vi "PDF_Interface_PDF Protokoll EPA1065_308 T90.vi"(8 "error in (no error)":errorcluster caption="Fehler (Eingang, kein Fehler)", 9 "ResultPictures":T1, 10 "SVGraph Referenz":refnum<vi>, 11 "Save PDF File Path":path) -> (0 "error out":errorcluster caption="Fehler (Ausgang)")   [LabVIEW 2020, in "EPA 1065.lvlib" / "T90 Test 1065-308.lvlib"]
uses:
  T90 Test 1065-308.lvlib
  Ergebnis.ctl
  PDF_Interface/PDF Interface Helper/PDFResultPictures.ctl
  Sprachverwaltung/FGV Aktion Tabelle zerlegen.ctl
  Aktion FGV T90.ctl
  Seiten/FT-IR/FGV FT-IR Gasliste Aktionen.ctl
  Seiten/FT-IR/FGV FT-IR Aktionen.ctl
  Seiten/System Einstellungen V2/Aktioen FGV System Konstanten.ctl
  PDF_Interface/PDF Protokoll Standard Kopf Optionen.ctl
  Visualisierungs Elemente/Auswahlfeld.ctl
  PDF_Interface/PDF Protokoll Standard Kopf Gasflasche Auswahl.ctl
  Aktion FGV Datenmanagment.ctl
  PDF_Interface/PDF Interface Helper/PDFGraph.ctl
  <vilib>/Simplicity AI/SAI_PDF_API/Classes/Context/Controls/SAI_PDF_Text Align.ctl
  PDF_Interface/PDF Interface Helper/PDFCommentPosition.ctl
  PDF_Interface/PDF Interface Helper/PDFPageBreak.ctl
  <vilib>/Simplicity AI/SAI_PDF_API/Classes/Context/Controls/SAI_PDF_PDF Details.ctl
  PDF_Interface/PDF Interface Helper/PDFContentType.ctl
  PDF_Interface/PDF Interface Helper/PDFTableContentType.ctl
  PDF_Interface/PDF Interface Helper/PDFResults.ctl
  PDF_Interface/PDF Interface Helper/PDFTablePictures.ctl
  PDF_Interface/PDF Interface Helper/PDFBemerkung.ctl
  <vilib>/Simplicity AI/SAI_PDF_API/Classes/Context/Controls/SAI_PDF_Font.ctl
  <vilib>/Simplicity AI/SAI_PDF_API/Classes/Context/Controls/SAI_PDF_Font Encoding.ctl
  Allgemein/allgemeine Sub-VIs.lvlib
  Seiten/FT-IR/FT-IR.lvlib
  Seiten/System Einstellungen V2/System Einstellungen V2.lvlib
  Sprachverwaltung/Sprachverwaltung.lvlib
  PDF_Interface/PDF Interface.lvlib
  PDF_Interface/PDF Interface Helper/PDF Interface Helper.lvlib
  <vilib>/Simplicity AI/SAI_PDF_API/Classes/Context/Context.lvclass
  Linearisierung V2/Protokoll/Protokoll.lvlib
panel:
  out "Frequenz 2":string
  out "Frequenz 1":string
  out "Versa Serial number:":string caption="Seriennummer:"
  out "Anlage:":string
  out "Methode (Recipe):":string
  out "Date & Time:":string caption="Datum & Uhrzeit:"
  out "Accuracy:":string caption="Genauigkeit:"
  out "Gas Bottle Nr.:":string caption="Gasflaschen Nr.:"
  out "Ergebnis 4":T2
  out "Ergebnis 3":T2
  out "Ergebnis 2":T2
  out "Ergebnis 1":T2
  out "Averaged T90-T10 2":string caption="gemittelter T90-T10"
  out "Averaged T10-T90 2":string caption="gemittelter T10-T90"
  out "Ergebnis x5 (T90 T10)":string caption="Mean T10-T90"
  out "Ergebnis x5 (T10 T90)":string caption="Mean T10-T90"
  out "Averaged T90-T10":string caption="gemittelter T90-T10"
  out "Averaged T10-T90":string caption="gemittelter T10-T90"
  out "T90 Result":waveform(sgl)(graph) caption="T90"
  out "Tabelle":string[][](table)
  out "Ergebnis:":string
  out "Konzentration:":string
  out "Komponente:":string
  out "Bearbeiter:":string caption="Editor:"
  out "Serial number:":string caption="Seriennummer:"
  out "Messgerät:":string
  # "T90 EPA § 1065.308"
  # "Grenzen"
  # "Ergebnis"
  # "s"
  # ">5"
  # "s"
  # ">5"
  # "s"
  # "<10s"
  # "s"
  # "<10s"
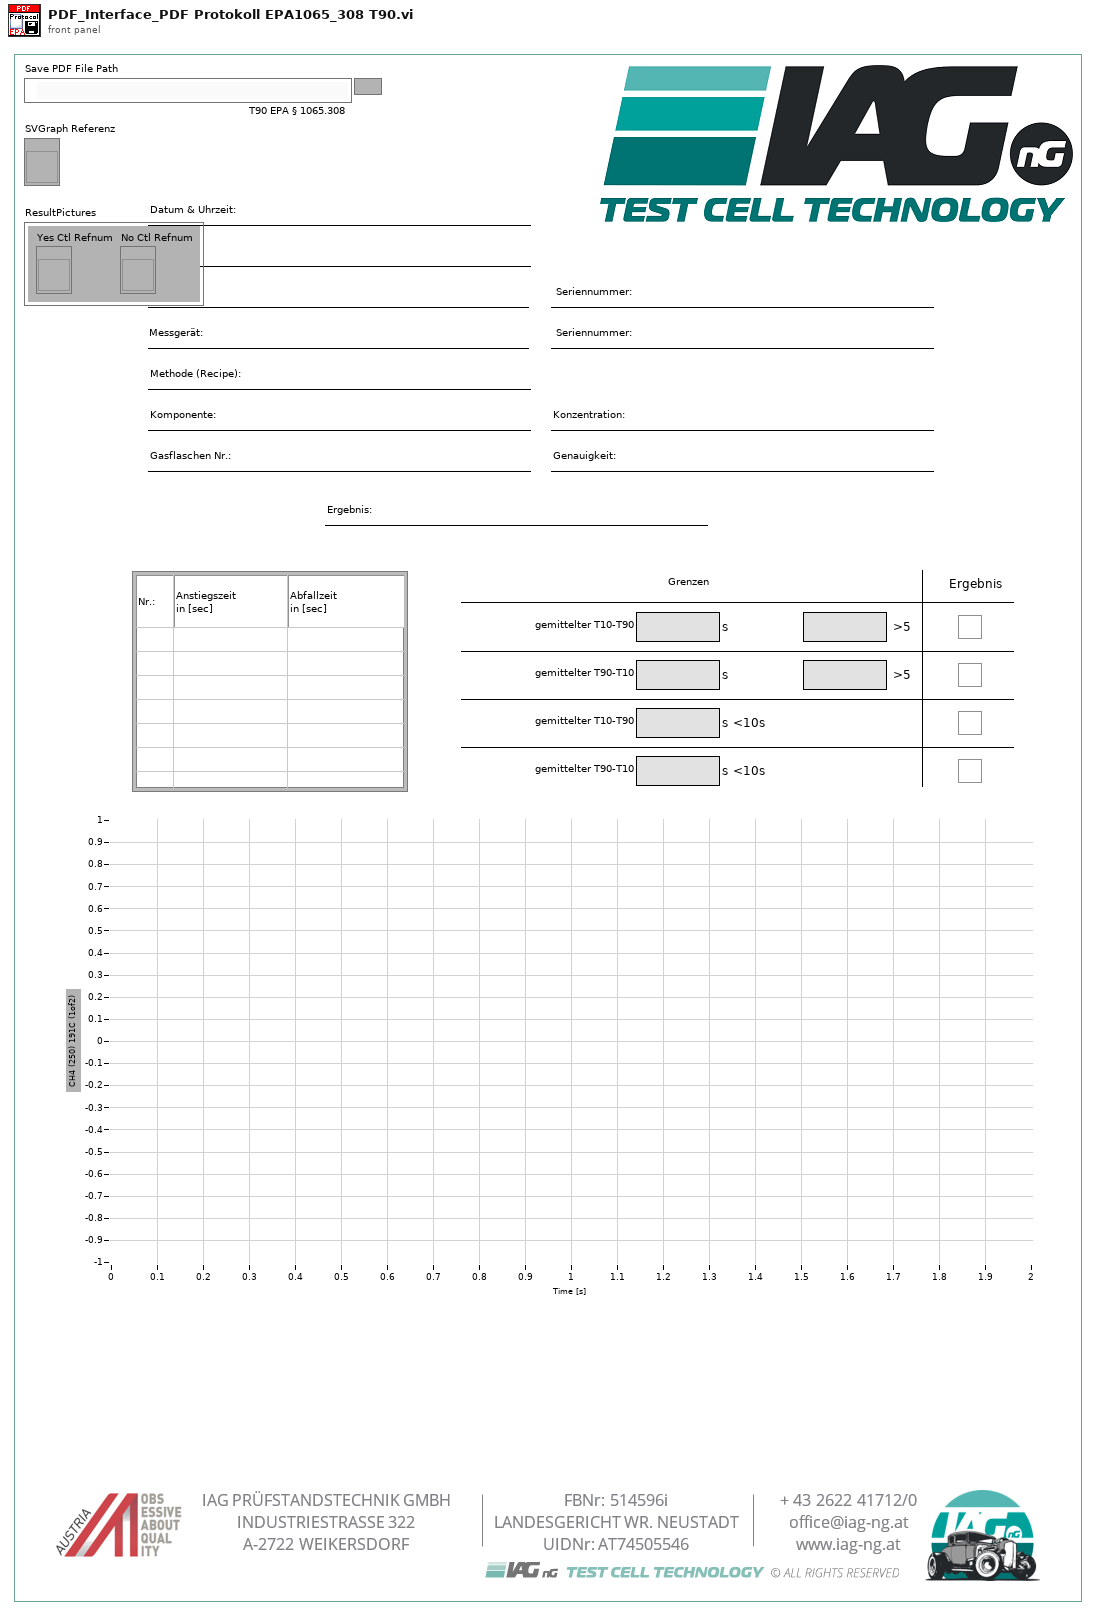
[diagram p1: front panel]
types:
  T1 = typedef "PDF Interface.lvlib/PDF Interface Helper.lvlib/PDFResultPictures.ctl" = cluster{"Yes Ctl Refnum":refnum<vi>, "No Ctl Refnum":refnum<vi>}
  T2 = typedef "EPA 1065.lvlib/T90 Test 1065-308.lvlib/Ergebnis.ctl" = bool
  T3 = typedef "Sprachverwaltung.lvlib/FGV Aktion Tabelle zerlegen.ctl" = enum16{"laden", "vereinzeln", "speichern"}
  T4 = typedef "PDF Interface.lvlib/PDF Protokoll Standard Kopf Gasflasche Auswahl.ctl" = cluster{"Gasflaschen Name":string, "Gasflaschen Nummer":string, "Gasnummer Index":i32}
  T5 = typedef "Auswahlfeld.ctl" = u16
  T6 = typedef "PDF Interface.lvlib/PDF Protokoll Standard Kopf Optionen.ctl" = cluster{"Analysator":bool, "FT-IR Rezept":bool, "Gasteiler":bool, "Gas Komponente":bool, "Gas Flasche":bool, "LIN Protokoll":bool, "Operator":bool}
  T7 = typedef "System Einstellungen V2.lvlib/Aktioen FGV System Konstanten.ctl" = enum16{"lesen", "laden", "speichern", "Sprache"}
  T8 = typedef "FT-IR.lvlib/FGV FT-IR Aktionen.ctl" = enum16{"lesen", "NOG setzen", "NOS setzen", "Initialisieren", "speichern", "ALLES setzen", "FT-IR Spektrum loggen", "Komm Stoppen", "Spektrum LogKonfig"}
  T9 = typedef "FT-IR.lvlib/FGV FT-IR Gasliste Aktionen.ctl" = enum16{"lesen", "Gasliste FT-IR", "Gasliste ausgelesen", "laden", "speichern", "löschen"}
  T10 = typedef "EPA 1065.lvlib/T90 Test 1065-308.lvlib/Aktion FGV T90.ctl" = enum16{"lesen", "Konfig Daten", "speichern", "laden", "T90 aktiv", "T90 inaktiv", "Ext. Ventil aktivieren", "Ext. Ventil deaktivieren", "N2 spülen aktiv", "N2 spülen inaktiv", "Ergebnis Textfile"}
  T11 = typedef "EPA 1065.lvlib/T90 Test 1065-308.lvlib/Aktion FGV Datenmanagment.ctl" = enum16{"init", "lesen", "Istwerte schreiben", "höchsten Peak setzen", "Auswerten", "Grenzen setzen", "Sollwert ändern", "Rise T10", "Rise T90", "Fall T90", "Fall T10", "Bit löschen", "Umschaltzeitpunkt"}
  T12 = typedef "PDF Interface.lvlib/PDF Interface Helper.lvlib/PDFBemerkung.ctl" = cluster{"Bemerkung Text":string, "Align (Left)":T13, "Add Line Feeds (F:No)":bool, "Font":T14}
  T13 = typedef "SAI_PDF_Toolkit.lvlib/Context.lvclass/SAI_PDF_Text Align.ctl" = i32
  T14 = typedef "SAI_PDF_Toolkit.lvlib/Context.lvclass/SAI_PDF_Font.ctl" = cluster{"Font":string, "Size":i32, "Colour":u32, "Bold":bool, "Italic":bool, "Underline":bool, "Strikethrough":bool, "Font Encoding":T15}
  T15 = typedef "SAI_PDF_Toolkit.lvlib/Context.lvclass/SAI_PDF_Font Encoding.ctl" = enum16{"Cp1252, WinANSI", "IdentityH", "IdentityV", "Cp1250", "Cp1257", "MacRoman"}
  T16 = typedef "PDF Interface.lvlib/PDF Interface Helper.lvlib/PDFContentType.ctl" = cluster{"Titel":string, "Header Table":string[][], "Table Array":T17[], "Bemerkungen":T12[]}
  T17 = typedef "PDF Interface.lvlib/PDF Interface Helper.lvlib/PDFTableContentType.ctl" = cluster{"TableHeader":string[], "Table":string[][], "Relative Column Widths (%)":sgl[], "Results":T18, "PositionBemerkung":T19, "PageBreak":T20, "TablePictures":T21, "Horizontal Align":i32}
  T18 = typedef "PDF Interface.lvlib/PDF Interface Helper.lvlib/PDFResults.ctl" = cluster{"Results":cluster{"Result Text":string, "Result":bool}[], "ResultPictures":T1, "use Pictures":bool, "Image Scale (%)":sgl, "Autoscale? (T)":bool, "Horizontal Align":i32, "Position":i32}
  T19 = typedef "PDF Interface.lvlib/PDF Interface Helper.lvlib/PDFCommentPosition.ctl" = enum16{"before", "after"}
  T20 = typedef "PDF Interface.lvlib/PDF Interface Helper.lvlib/PDFPageBreak.ctl" = enum16{"none", "before", "after", "after comment"}
  T21 = typedef "PDF Interface.lvlib/PDF Interface Helper.lvlib/PDFTablePictures.ctl" = cluster{"Ctl Refnum In":refnum<vi>[], "RowOrColumn":enum16{"Row", "Column"}, "IndexToInsert":u16, "Image Scale (%)":sgl[], "Autoscale? (T)":bool[], "Horizontal Align":i32}
  T22 = typedef "SAI_PDF_Toolkit.lvlib/Context.lvclass/SAI_PDF_PDF Details.ctl" = cluster{"Title":string, "Subject":string, "Keywords":string, "Author":string, "Creator":string}
  T23 = cluster{"Header Footer Text Cluster":cluster{"Header Text":string, "Footer Text":string, "Time":string, "Page Number":string}, "PDF Details":T22}
  T24 = typedef "EPA 1065.lvlib/T90 Test 1065-308.lvlib/T90 Konfig Daten.ctl" = cluster{"Bearbeiter:":string, "Komponente:":u16, "Gasflaschen Nr.:":string, "Accuracy":dbl, "Sollwert":dbl, "Modus":T25, "Abschaltzeit:":dbl, "Abweichung:":dbl, "Pfad:":path, "Textname:":string, "CG Aufschaltzeit:":dbl, "Einheit":string, "N2 Aufschaltzeit:":dbl, "Analysator":T26, "Gasflasche":T27, "Konfig Gasflasche":T28, "Frequency:":T29}
  T25 = typedef "EPA 1065.lvlib/T90 Test 1065-308.lvlib/Modus.ctl" = u16
  T26 = typedef "System Einstellungen V2.lvlib/Analysatoren.ctl" = string
  T27 = typedef "System Einstellungen V2.lvlib/Gasflasche Auswahl.ctl" = u16
  T28 = typedef "System Einstellungen V2.lvlib/Konfig Gasflasche.ctl" = bool
  T29 = typedef "EPA 1065.lvlib/T90 Test 1065-308.lvlib/Frequenz.ctl" = u16
  T30 = typedef "String - Ausgabefeld.ctl" = string
  T31 = cluster{"Header Size":i32, "Column Ratio left":sgl[]}
  T32 = cluster{"Modell":string, "ProjektNummer":string, "Software Version":string, "Seriennummer":string}
  T33 = typedef "EPA 1065.lvlib/T90 Test 1065-308.lvlib/Datencluster.ctl" = cluster{"Höchster Peak":T34, "T10 Grenzwert":T34, "T90 Grenzwert":T34, "Rise Times":dbl[], "Fall Times":dbl[], "RiseTime gemittelt":T34, "FallTime gemittelt":T34, "Zeitstempel":timestamp[], "Rise T10":bool, "Rise T90":bool, "Fall T10":bool, "Fall T90":bool, "RiseTime >5":bool, "Falltime >5":bool, "RiseTime <10":bool, "Falltime <10":bool, "T0-T90":dbl[], "T100-T10":dbl[]}
  T34 = typedef "Zahlen-Eingabefeld.ctl" = sgl
  T35 = typedef "PDF Interface.lvlib/PDF Interface Helper.lvlib/PDFGraph.ctl" = cluster{"GraphCtl Refnum":refnum<vi>, "Wrap Text (F:No)":bool, "Hide Grid (F:No)":bool, "Scale (100%)":sgl, "Align (Left)":T13, "PositionBemerkung":T19, "PageBreak":T20}
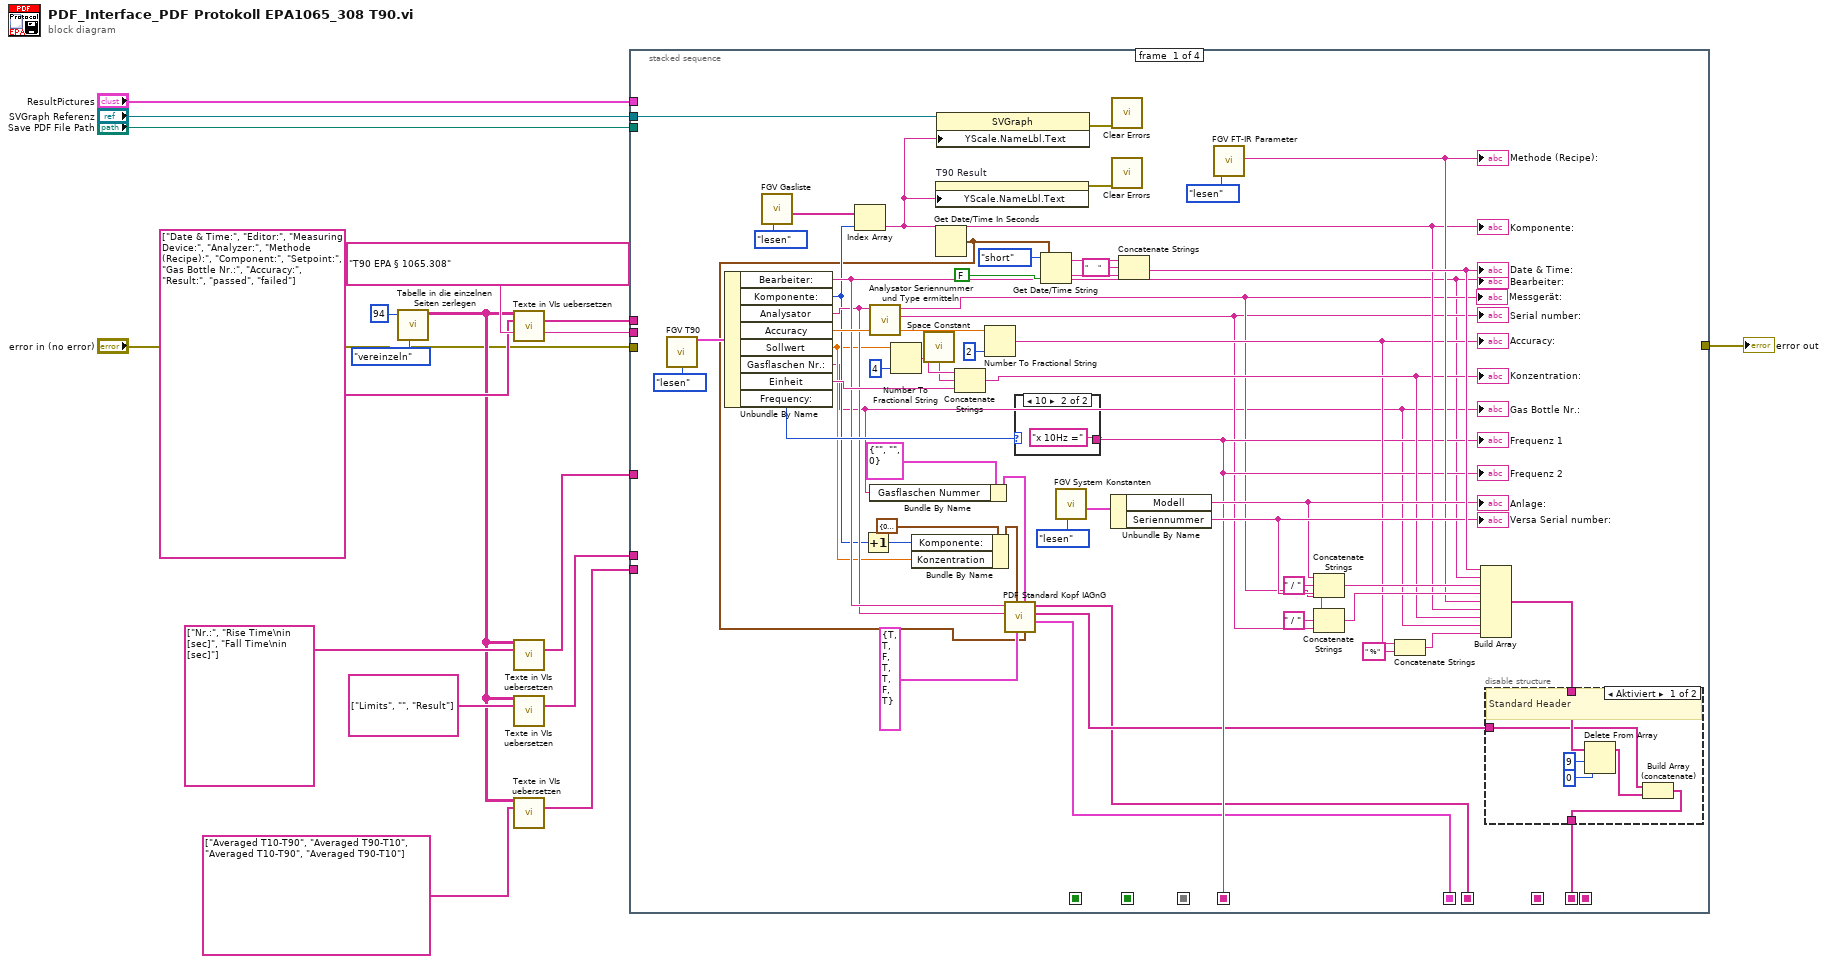
[diagram p0: block diagram]
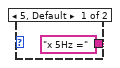
[diagram p3: hidden frame]
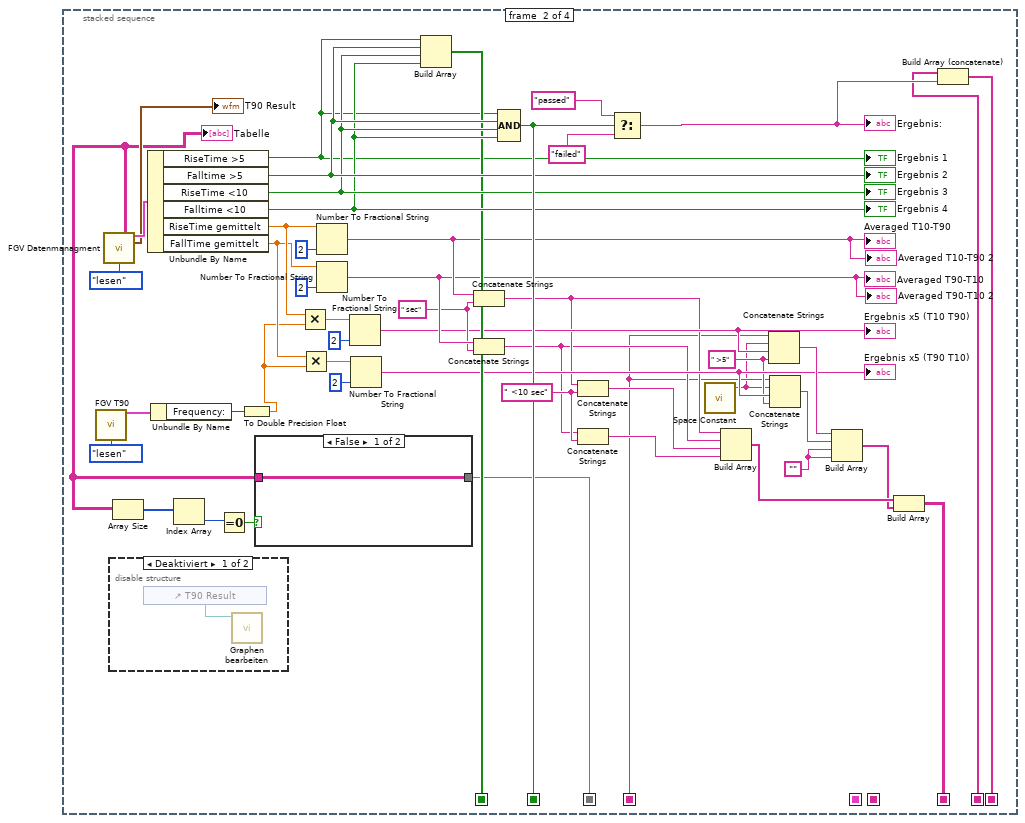
[diagram p4: hidden frame]
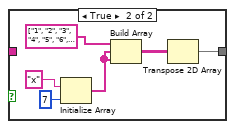
[diagram p5: hidden frame]
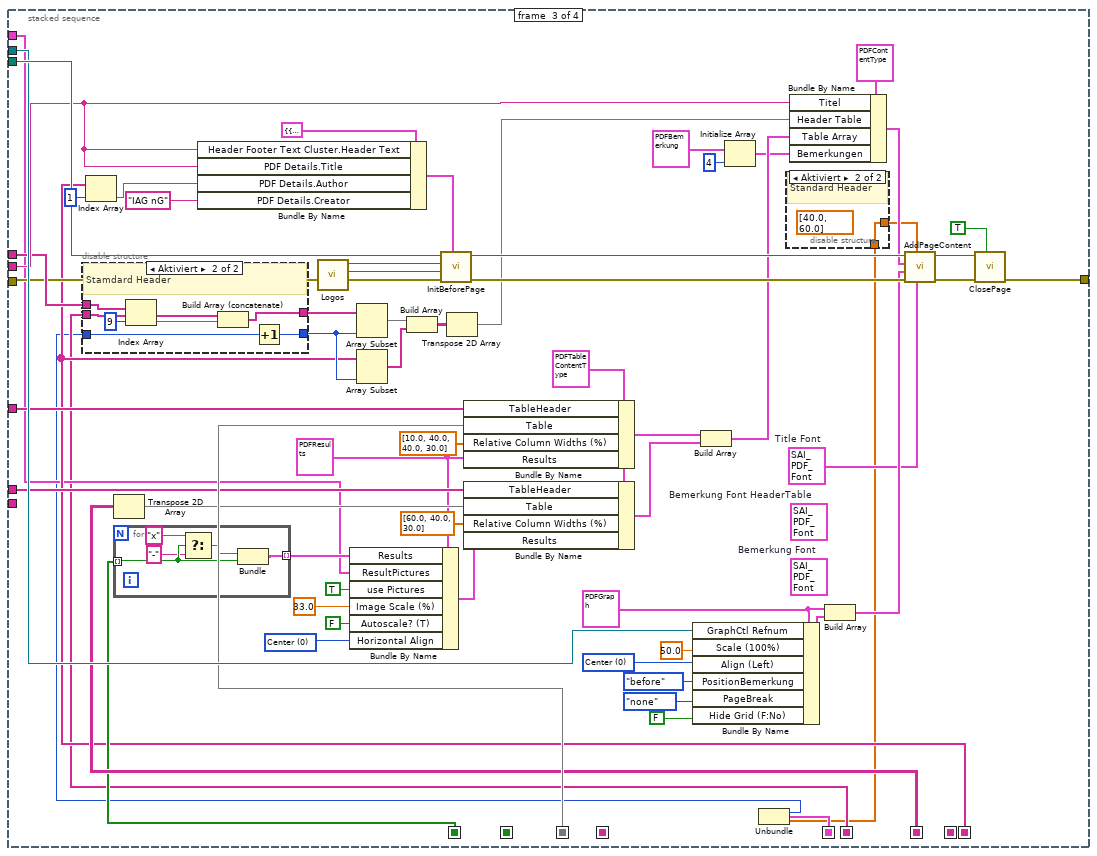
[diagram p7: hidden frame]
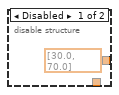
[diagram p8: hidden frame]
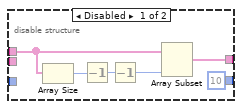
[diagram p9: hidden frame]
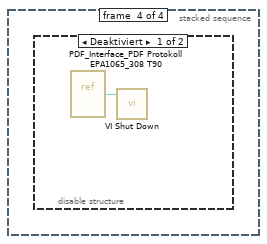
[diagram p10: hidden frame]
diagram:
  n1 = call "Tabelle in die einzelnen Seiten zerlegen.vi"("Aktion"=FGV_Aktion_Tabelle_zerlegen."vereinzeln", "Index (Seite)"=94) -> ("Sprachliste"=w8:string[][])  [unwired: 7 in, 2 out]
  n2 = call "Texte in VIs uebersetzen.vi"("Sprachliste"=w8, "String-Array zum Übersetzen"=string[] ["Date & Time:", "Editor:", "Measuring Device:", "Analyzer:", "Methode (Recipe):", "Component:", "Setpoint:", "Gas Bottle Nr.:", "Accuracy:", "Result:", "passed", "failed"], "String zum Übersetzen"="T90 EPA § 1065.308") -> ("String-Array zum Übersetzen"=w13:string[], "String zum Übersetzen"=w14:string)  [unwired: 8 in, 3 out]
  n3 = call "Texte in VIs uebersetzen.vi"("Sprachliste"=w8, "String-Array zum Übersetzen"=string[] ["Nr.:", "Rise Time\nin [sec]", "Fall Time\nin [sec]"]) -> ("String-Array zum Übersetzen"=w6:string[])  [unwired: 9 in, 4 out]
  n4 = call "Texte in VIs uebersetzen.vi"("Sprachliste"=w8, "String-Array zum Übersetzen"=string[] ["Limits", "", "Result"]) -> ("String-Array zum Übersetzen"=w5:string[])  [unwired: 9 in, 4 out]
  n5 = call "Texte in VIs uebersetzen.vi"("Sprachliste"=w8, "String-Array zum Übersetzen"=string[] ["Averaged T10-T90", "Averaged T90-T10", "Averaged T10-T90", "Averaged T90-T10"]) -> ("String-Array zum Übersetzen"=w4:string[])  [unwired: 9 in, 4 out]
  n6 = stacked-sequence {
    seq-local: [_ w86 _ _] -> [_ _ w166 _]
    seq-local: [_ w115 _ _] -> [_ _ _ _]
    seq-local: [_ w111 _ _] -> [_ _ w160 _]
    seq-local: [w23 _ _ _] -> [_ w109 _ _]
    seq-local: [_ w108 _ _] -> [_ _ w155 _]
    seq-local: [_ w91 _ _] -> [_ _ w161 _]
    seq-local: [w38 _ _ _] -> [_ w85 _ _]
    seq-local: [w22 _ _ _] -> [_ _ w144 _]
    seq-local: [w21 _ _ _] -> [_ _ w143 _]
    tunnel: w14 -> [_ _ w170 _]
    tunnel: w13 -> [_ _ w169 _]
    tunnel: "Save PDF File Path" -> [_ _ w172 _]
    tunnel: "SVGraph Referenz" -> [w54 _ w171 _]
    tunnel: w6 -> [_ _ w165 _]
    tunnel: w5 -> [_ _ w163 _]
    tunnel: w4 -> [_ _ _ _]
    tunnel: "error in (no error)" -> [_ _ w168 _]
    tunnel: [_ _ w167 _] -> w2
    tunnel: "ResultPictures" -> [_ _ w150 _]
    frame #0 {
      n7 = call "FGV T90.vi"("Aktion"=Aktion_FGV_T90."lesen") -> ("T90 Konfig Daten"=w67:T24)  [unwired: 9 in, 5 out]
      n8 = Unbundle By Name(w67) -> ("Bearbeiter:"=w34:string, "Komponente:"=w30:u16, "Analysator"=w33:T26, "Accuracy"=w63:dbl, "Sollwert"=w29:dbl, "Gasflaschen Nr.:"=w26:string, "Einheit"=w58:string, "Frequency:"=w55:T29)
      "Gas Bottle Nr.:" <- w26
      "Bearbeiter:" <- w34
      n9 = call "FGV Gasliste.vi"("Aktionen"=FGV_FT-IR_Gasliste_Aktionen."lesen") -> ("Aktuelle Gasliste gesamt"=w65:T30[])  [unwired: 8 in, 2 out]
      n10 = Index Array(array=w65, index=w30) -> (element=w43:T30)
      "Komponente:" <- w43
      n11 = Increment(x=w30) -> (x+1=w20:u16)
      n12 = call "Analysator Seriennummer und Type ermitteln.vi"("Analysator"=w33) -> ("Type"=w36:string, "Name für Protokoll"=w37:string)  [unwired: 8 in, 1 out]
      "Messgerät:" <- w37
      "Serial number:" <- w36
      n13 = Bundle By Name(cluster=T4 {"Gasflaschen Name"="", "Gasflaschen Nummer"="", "Gasnummer Index"=0} ("Gaschflasche Cluster"), "Gasflaschen Nummer"=w26) -> (w27:T4)
      n14 = Number To Fractional String(number=w29, precision (6)=i16 4 ("Genauigkeit (6)")) -> (F-format string=w60:string)  [unwired: 2 in]
      n15 = Bundle By Name(cluster=cluster{"Komponente:":T5, "Konzentration":dbl} {"Komponente:"=0, "Konzentration"=0.0} ("Gas Komponente"), "Komponente:"=w20, "Konzentration"=w29) -> (w31:cluster{"Komponente:":T5, "Konzentration":dbl})
      n16 = call <vilib>:"Space Constant.vi"() -> ("String"=w59:string)
      n17 = property on="T90 Result" class="SVGraph (strikt)"("YScale.NameLbl.Text"=w43) -> (error out=w53:errorcluster)  [unwired: 2 in, 1 out]
      n18 = Get Date/Time In Seconds() -> (seconds since 1Jan1904=w19:timestamp)
      n19 = property class="SVGraph"(reference=w54, "YScale.NameLbl.Text"=w43) -> (error out=w52:errorcluster)  [unwired: 1 in, 1 out]
      n20 = Concatenate Strings(w60, w59, w58) -> (w42:string)
      "Konzentration:" <- w42
      n21 = Number To Fractional String(number=w63, precision (6)=i16 2 ("Genauigkeit (6)")) -> (F-format string=w41:string)  [unwired: 2 in]
      "Accuracy:" <- w41
      n22 = call "PDF Standard Kopf IAGnG.vi"("Zeitstempel"=w19, "Gaschflasche Cluster"=w27, "Oprtionen Cluster"=T6 {"Analysator"=TRUE, "FT-IR Rezept"=TRUE, "Gasteiler"=FALSE, "Gas Komponente"=TRUE, "Gas Flasche"=TRUE, "LIN Protokoll"=FALSE, "Operator"=TRUE}, "Gas Komponente"=w31, "Analysator"=w33, "Bearbeiter/in"=w34) -> ("Size Cluster"=w21:T31, "Header Values"=w24:T30[], "Header Labels"=w22:string[])  [unwired: 2 in, 1 out]
      n23 = case shown="10" w55 {
        tunnel: ["x 5Hz =" "x 10Hz ="] -> w38
        frame 5, Default {
        }
        frame 10 {
        }
      }
      "Frequenz 1" <- w38
      "Frequenz 2" <- w38
      n24 = Get Date/Time String(date format (0)=enum16{"short", "long", "abbreviated"}."short" ("Datumsformat (0)"), seconds (now)=w19, want seconds? (F)=FALSE ("Angabe von Sekunden? (F)")) -> (date string=w73:string, time string=w72:string)
      n25 = call "FGV System Konstanten.vi"("Aktionen"=Aktioen_FGV_System_Konstanten."lesen") -> ("Cluster out"=w56:T32)  [unwired: 6 in, 4 out]
      n26 = Unbundle By Name(w56) -> ("Modell"=w46:string, "Seriennummer"=w49:string)
      "Versa Serial number:" <- w49
      "Anlage:" <- w46
      n27 = call <vilib>:"Clear Errors.vi"("error in (no error)"=w52) -> ()  [unwired: 5 in, 2 out]
      n28 = call <vilib>:"Clear Errors.vi"("error in (no error)"=w53) -> ()  [unwired: 5 in, 2 out]
      n29 = Concatenate Strings(w73, "     " ("String"), w72) -> (w51:string)
      "Date & Time:" <- w51
      n30 = call "FGV FT-IR Parameter.vi"("Aktion"=FGV_FT-IR_Aktionen."lesen") -> ("Current Recipe"=w44:string)  [unwired: 11 in, 7 out]
      "Methode (Recipe):" <- w44
      n31 = Concatenate Strings(w46, " / " ("String"), w49) -> (w48:string)
      n32 = Concatenate Strings(w37, " / " ("String"), w36) -> (w45:string)
      n33 = Concatenate Strings(w41, " %" ("String")) -> (w39:string)
      n34 = Build Array(w51, w34, w48, w45, w44, w43, w42, w26, w39) -> (w25:T30[])
      n35 = disable-structure shown="Aktiviert" {
        disable-tunnel: w25 -> [w79 w80]
        disable-tunnel: w24 -> [w75 _]
        disable-tunnel: [w74 w80] -> w23
        frame Enabled {
          # "Standard Header"
          n36 = Delete From Array(array=w79, length=9 ("Länge"), index=0 ("Index")) -> (array with subset deleted=w76:T30[])  [unwired: 1 out]
          n37 = Build Array (concatenate)(w75, w76) -> (w74:T30[])
        }
        frame Disabled {
        }
      }
    }
    frame #1 {
      w94 = ""
      w98 = " <10 sec" ("String")
      w101 = " >5" ("String")
      w105 = " sec"
      n38 = call "FGV T90.vi"("Aktion"=Aktion_FGV_T90."lesen") -> ("T90 Konfig Daten"=w118:T24)  [unwired: 9 in, 5 out]
      n39 = call "FGV Datenmanagment.vi"("Aktion"=Aktion_FGV_Datenmanagment."lesen") -> ("Ergebnistabelle"=w87:string[][], "Daten"=w131:T33, "T90 Signalverlauf"=→"T90 Result":waveform(sgl))  [unwired: 7 in, 5 out]
      "Tabelle" <- w87
      n40 = disable-structure shown="Deaktiviert" {
        frame Disabled {
          n41 = control-ref of="T90 Result"() -> (w140:refnum<vi>)
          n42 = call "Graphen bearbeiten.vi"("T90 Result"=w140) -> ()  [unwired: 10 in, 1 out]
        }
        frame Enabled {
        }
      }
      n43 = Array Size(array=w87) -> (size(s)=w90:i32[])
      n44 = Unbundle By Name(w131) -> ("RiseTime >5"=w83:bool, "Falltime >5"=w114:bool, "RiseTime <10"=w113:bool, "Falltime <10"=w112:bool, "RiseTime gemittelt"=w124:T34, "FallTime gemittelt"=w123:T34)
      "Ergebnis 4" <- w112
      "Ergebnis 3" <- w113
      "Ergebnis 2" <- w114
      "Ergebnis 1" <- w83
      n45 = Unbundle By Name(w118) -> ("Frequency:"=w117:T29)
      n46 = Index Array(array=w90) -> (element=w89:i32)  [unwired: 1 in]
      n47 = Equal To 0?(x=w89) -> (x = 0?=w88:bool)
      n48 = To Double Precision Float(number=w117) -> (double precision float=w116:dbl)
      n49 = case shown="False" w88 {
        tunnel: [w133 w134] -> w86
        tunnel: w87 -> [w133 _]
        frame False {
        }
        frame True {
          n50 = Initialize Array("x", 7 ("Dimensionsgröße")) -> (w136:string[])
          n51 = Build Array(string[] ["1", "2", "3", "4", "5", "6", "7"], w136, w136) -> (w135:string[][])
          n52 = Transpose 2D Array(2D array=w135) -> (transposed array=w134:string[][])
        }
      }
      n53 = Multiply(x=w124, y=w116) -> (x*y=w128:dbl)
      n54 = Multiply(x=w123, y=w116) -> (x*y=w127:dbl)
      n55 = Number To Fractional String(number=w124, precision (6)=i16 2 ("Genauigkeit (6)")) -> (F-format string=w107:string)  [unwired: 2 in]
      "Averaged T10-T90 2" <- w107
      "Averaged T10-T90" <- w107
      n56 = Number To Fractional String(number=w123, precision (6)=i16 2 ("Genauigkeit (6)")) -> (F-format string=w106:string)  [unwired: 2 in]
      "Averaged T90-T10 2" <- w106
      "Averaged T90-T10" <- w106
      n57 = Number To Fractional String(number=w128, precision (6)=i16 2 ("Genauigkeit (6)")) -> (F-format string=w104:string)  [unwired: 2 in]
      "Ergebnis x5 (T10 T90)" <- w104
      n58 = Number To Fractional String(number=w127, precision (6)=i16 2 ("Genauigkeit (6)")) -> (F-format string=w102:string)  [unwired: 2 in]
      "Ergebnis x5 (T90 T10)" <- w102
      n59 = Build Array(w83, w114, w113, w112) -> (w111:bool[])
      n60 = Concatenate Strings(w107, w105) -> (w99:string)
      n61 = Concatenate Strings(w106, w105) -> (w97:string)
      n62 = Compound Arithmetic op=AND ("Mehrfacharithmetik")(w83, w114, w113, w112) -> (w115:bool)
      n63 = Concatenate Strings(w99, w98) -> (w96:string)
      n64 = Concatenate Strings(w97, w98) -> (w95:string)
      n65 = Select(t="passed", s=w115, f="failed") -> (s? t:f=w110:string)
      "Ergebnis:" <- w110
      n66 = call <vilib>:"Space Constant.vi"() -> ("String"=w84:string)
      n67 = Build Array(w99, w97, w96, w95) -> (w93:string[])
      n68 = Concatenate Strings(w85, w84, w104, w101) -> (w103:string)
      n69 = Concatenate Strings(w85, w84, w102, w101) -> (w100:string)
      n70 = Build Array(w103, w100, w94, w94) -> (w92:string[])
      n71 = Build Array(w93, w92) -> (w91:string[][])
      n72 = Build Array (concatenate)(w109, w110) -> (w108:T30[])
    }
    frame #2 {
      w147 = T13 0 items=["Center", "Justified", "Justified All", "Left", "Right"] ("Align (Left)")
      w152 = T18 {"Results"=[], "ResultPictures"={"Yes Ctl Refnum"=refnum, "No Ctl Refnum"=refnum}, "use Pictures"=FALSE, "Image Scale (%)"=100.0, "Autoscale? (T)"=TRUE, "Horizontal Align"=3, "Position"=0} ("Results")
      w154 = T17 {"TableHeader"=[], "Table"=[], "Relative Column Widths (%)"=[], "Results"={"Results"=[], "ResultPictures"={"Yes Ctl Refnum"=refnum, "No Ctl Refnum"=refnum}, "use Pictures"=FALSE, "Image Scale (%)"=100.0, "Autoscale? (T)"=TRUE, "Horizontal Align"=3, "Position"=0}, "PositionBemerkung"=enum."before", "PageBreak"=enum."none", "TablePictures"={"Ctl Refnum In"=[], "RowOrColumn"=enum."Row", "IndexToInsert"=0, "Image Scale (%)"=[], "Autoscale? (T)"=[], "Horizontal Align"=0}, "Horizontal Align"=0} ("Table Array")
      (unwired) T14 {"Font"="Arial", "Size"=12, "Colour"=16711680, "Bold"=TRUE, "Italic"=TRUE, "Underline"=FALSE, "Strikethrough"=FALSE, "Font Encoding"=enum."Cp1252, WinANSI"}  # Bemerkung Font HeaderTable
      (unwired) T14 {"Font"="Arial", "Size"=12, "Colour"=0, "Bold"=TRUE, "Italic"=TRUE, "Underline"=FALSE, "Strikethrough"=FALSE, "Font Encoding"=enum."Cp1252, WinANSI"}  # Bemerkung Font
      w173 = T14 {"Font"="Arial", "Size"=26, "Colour"=0, "Bold"=TRUE, "Italic"=FALSE, "Underline"=TRUE, "Strikethrough"=FALSE, "Font Encoding"=enum."Cp1252, WinANSI"}  # Title Font
      w178 = T13 0 items=["Center", "Justified", "Justified All", "Left", "Right"] ("Align (Left)")
      w159 = T35 {"GraphCtl Refnum"=refnum, "Wrap Text (F:No)"=FALSE, "Hide Grid (F:No)"=FALSE, "Scale (100%)"=100.0, "Align (Left)"=0, "PositionBemerkung"=enum."before", "PageBreak"=enum."after comment"} ("Graph")
      n73 = Index Array(array=w155, index=1 ("Index")) -> (element=w156:T30)
      n74 = Transpose 2D Array(2D array=w161) -> (transposed array=w158:string[][])
      n75 = for {
        tunnel: w160 -> [w223] mode=indexing
        tunnel: [w224] -> w151 mode=indexing
        n76 = Select(t="x", s=w223, f="-") -> (s? t:f=w220:string)
        n77 = Bundle(w220, "Falltime <10"=w223) -> (w224:cluster{string, "Falltime <10":bool})  [unwired: 1 in]
      }
      n78 = Bundle By Name(cluster=T23 {"Header Footer Text Cluster"={"Header Text"="Protokoll XYZ", "Footer Text"="IAG nG", "Time"="<TIMESTAMP yyyy-MM-dd>", "Page Number"="Page <P> of <PT>"}, "PDF Details"={"Title"="Test PDF", "Subject"="Versa Tabasco", "Keywords"="", "Author"="RIW", "Creator"="IAG"}} ("Info"), "Header Footer Text Cluster.Header Text"=w170, "PDF Details.Title"=w170, "PDF Details.Author"=w156, "PDF Details.Creator"="IAG nG") -> (w195:T23)
      n79 = call "Logos.vi"() -> ("Footer Image File Path"=w203:path, "Header Image File Path"=w204:path)  [unwired: 8 in, 2 out]
      n80 = Bundle By Name(cluster=w152, "Results"=w151, "ResultPictures"=w150, "use Pictures"=TRUE, "Image Scale (%)"=sgl 33.0, "Autoscale? (T)"=FALSE, "Horizontal Align"=w147) -> (w153:T18)
      n81 = call "InitBeforePage.vi"("Info"=w195, "Fehler (Eingang, kein Fehler)"=w168, "Footer Image File Path"=w203, "Header Image File Path"=w204, "Path (Dialog if Empty)"=w172) -> ("Fehler (Ausgang)"=w202:errorcluster, "Context (Ausgang)"=w201:refnum<class "Context.lvclass">)  [unwired: 5 in]
      n82 = Bundle By Name(cluster=w154, "TableHeader"=w165, "Table"=w166, "Relative Column Widths (%)"=sgl[] [10.0, 40.0, 40.0, 30.0], "Results"=w152) -> (w187:T17)
      n83 = Bundle By Name(cluster=w154, "TableHeader"=w163, "Table"=w158, "Relative Column Widths (%)"=sgl[] [60.0, 40.0, 30.0], "Results"=w153) -> (w164:T17)
      n84 = Bundle By Name(cluster=w159, "GraphCtl Refnum"=w171, "Scale (100%)"=sgl 50.0, "Align (Left)"=w178, "PositionBemerkung"=PDFCommentPosition."before", "PageBreak"=PDFPageBreak."none", "Hide Grid (F:No)"=FALSE) -> (w182:T35)
      n85 = Build Array(w187, w164) -> (w186:T17[])
      n86 = Initialize Array(T12 {"Bemerkung Text"="", "Align (Left)"=0, "Add Line Feeds (F:No)"=FALSE, "Font"={"Font"="Arial", "Size"=10, "Colour"=0, "Bold"=FALSE, "Italic"=FALSE, "Underline"=FALSE, "Strikethrough"=FALSE, "Font Encoding"=enum."Cp1252, WinANSI"}} ("Bemerkung"), 4 ("Dimensionsgröße")) -> (w175:T12[])
      n87 = Unbundle(w143) -> ("Header Size"=w142:i32, "Column Ratio left"=w141:sgl[])
      n88 = disable-structure shown="Aktiviert" {
        disable-tunnel: [w209 w214] -> w190
        disable-tunnel: [10 ("Länge") w218] -> w189
        disable-tunnel: w169 -> [w207 w216]
        disable-tunnel: w144 -> [_ w217]
        disable-tunnel: w142 -> [_ w219]
        frame Disabled {
          n89 = Array Size(array=w207) -> (size(s)=w212:i32)
          n90 = Decrement(x=w212) -> (x-1=w211:i32)
          n91 = Decrement(x=w211) -> (x-1=w210:i32)
          n92 = Array Subset(array=w207, length=w210) -> (w209:string[])  [unwired: 1 in]
        }
        frame Enabled {
          # "Stamdard Header"
          n93 = Index Array(array=w216, index=9 ("Index")) -> (element=w215:string)
          n94 = Build Array (concatenate)(w217, w215) -> (w214:string[])
          n95 = Increment(x=w219) -> (x+1=w218:i32)
        }
      }
      n96 = Array Subset(array=w190, length=w189) -> (w193:string[])  [unwired: 1 in]
      n97 = Array Subset(array=w155, length=w189) -> (w192:T30[])  [unwired: 1 in]
      n98 = Build Array(w193, w192) -> (w191:T30[][])
      n99 = Transpose 2D Array(2D array=w191) -> (transposed array=w183:T30[][])
      n100 = disable-structure shown="Aktiviert" {
        disable-tunnel: [sgl[] [30.0, 70.0] ("Column Ratio left") w206] -> w184
        disable-tunnel: w141 -> [_ w206]
        frame Disabled {
        }
        frame Enabled {
          (unwired) sgl[] [40.0, 60.0] ("Column Ratio left")
          # "Standard Header"
        }
      }
      n101 = Bundle By Name(cluster=T16 {"Titel"="Test mit Graph und Results PDF", "Header Table"=[["Murks:", "4711"], ["HolyShit:", "0815"]], "Table Array"=[{"TableHeader"=["Soll\nppm/%", "Ist\nppm/%", "Fehler\n%", "Toleranz\n%", "Ergebnis"], "Table"=[["aaa", "bbb", "ccc", "ddd"], ["111", "222", "333", "444"], ["sss", "fff", "kkk", "xxx"], ["6.5", "11.13", "19.2", "4"], ["1111", "1212", "777", "888"]], "Relative Column Widths (%)"=[22.5, 22.5, 22.5, 22.5, 10.0], "Results"={"Results"=[], "ResultPictures"={"Yes Ctl Refnum"=refnum, "No Ctl Refnum"=refnum}, "use Pictures"=FALSE, "Image Scale (%)"=100.0, "Autoscale? (T)"=TRUE, "Horizontal Align"=3, "Position"=0}, "PositionBemerkung"=enum."after", "PageBreak"=enum."none", "TablePictures"={"Ctl Refnum In"=[], "RowOrColumn"=enum."Row", "IndexToInsert"=0, "Image Scale (%)"=[], "Autoscale? (T)"=[], "Horizontal Align"=3}, "Horizontal Align"=3}, {"TableHeader"=["Soll\nppm/%", "Ist\nppm/%", "Fehler\n%", "Toleranz\n%", "Ergebnis"], "Table"=[["aaa", "bbb", "ccc", "ddd"], ["111", "222", "333", "444"], ["sss", "fff", "kkk", "xxx"], ["6.5", "11.13", "19.2", "4"], ["1111", "1212", "777", "888"]], "Relative Column Widths (%)"=[22.5, 22.5, 22.5, 22.5, 10.0], "Results"={"Results"=[], "ResultPictures"={"Yes Ctl Refnum"=refnum, "No Ctl Refnum"=refnum}, "use Pictures"=FALSE, "Image Scale (%)"=100.0, "Autoscale? (T)"=TRUE, "Horizontal Align"=3, "Position"=0}, "PositionBemerkung"=enum."before", "PageBreak"=enum."before", "TablePictures"={"Ctl Refnum In"=[], "RowOrColumn"=enum."Row", "IndexToInsert"=0, "Image Scale (%)"=[], "Autoscale? (T)"=[], "Horizontal Align"=3}, "Horizontal Align"=3}, {"TableHeader"=["Soll\nppm/%", "Ist\nppm/%", "Fehler\n%", "Toleranz\n%", "Ergebnis"], "Table"=[["aaa", "bbb", "ccc", "ddd"], ["111", "222", "333", "444"], ["sss", "fff", "kkk", "xxx"], ["6.5", "11.13", "19.2", "4"], ["1111", "1212", "777", "888"]], "Relative Column Widths (%)"=[22.5, 22.5, 22.5, 22.5, 10.0], "Results"={"Results"=[], "ResultPictures"={"Yes Ctl Refnum"=refnum, "No Ctl Refnum"=refnum}, "use Pictures"=FALSE, "Image Scale (%)"=100.0, "Autoscale? (T)"=TRUE, "Horizontal Align"=3, "Position"=0}, "PositionBemerkung"=enum."before", "PageBreak"=enum."before", "TablePictures"={"Ctl Refnum In"=[], "RowOrColumn"=enum."Row", "IndexToInsert"=0, "Image Scale (%)"=[], "Autoscale? (T)"=[], "Horizontal Align"=3}, "Horizontal Align"=3}, {"TableHeader"=["Soll\nppm/%", "Ist\nppm/%", "Fehler\n%", "Toleranz\n%", "Ergebnis"], "Table"=[["aaa", "bbb", "ccc", "ddd"], ["111", "222", "333", "444"], ["sss", "fff", "kkk", "xxx"], ["6.5", "11.13", "19.2", "4"], ["1111", "1212", "777", "888"]], "Relative Column Widths (%)"=[22.5, 22.5, 22.5, 22.5, 10.0], "Results"={"Results"=[], "ResultPictures"={"Yes Ctl Refnum"=refnum, "No Ctl Refnum"=refnum}, "use Pictures"=FALSE, "Image Scale (%)"=100.0, "Autoscale? (T)"=TRUE, "Horizontal Align"=3, "Position"=0}, "PositionBemerkung"=enum."before", "PageBreak"=enum."before", "TablePictures"={"Ctl Refnum In"=[], "RowOrColumn"=enum."Row", "IndexToInsert"=0, "Image Scale (%)"=[], "Autoscale? (T)"=[], "Horizontal Align"=3}, "Horizontal Align"=3}, {"TableHeader"=["Soll\nppm/%", "Ist\nppm/%", "Fehler\n%", "Toleranz\n%", "Ergebnis"], "Table"=[["aaa", "bbb", "ccc", "ddd"], ["111", "222", "333", "444"], ["sss", "fff", "kkk", "xxx"], ["6.5", "11.13", "19.2", "4"], ["1111", "1212", "777", "888"]], "Relative Column Widths (%)"=[22.5, 22.5, 22.5, 22.5, 10.0], "Results"={"Results"=[], "ResultPictures"={"Yes Ctl Refnum"=refnum, "No Ctl Refnum"=refnum}, "use Pictures"=FALSE, "Image Scale (%)"=100.0, "Autoscale? (T)"=TRUE, "Horizontal Align"=3, "Position"=0}, "PositionBemerkung"=enum."before", "PageBreak"=enum."before", "TablePictures"={"Ctl Refnum In"=[], "RowOrColumn"=enum."Row", "IndexToInsert"=0, "Image Scale (%)"=[], "Autoscale? (T)"=[], "Horizontal Align"=3}, "Horizontal Align"=3}], "Bemerkungen"=[{"Bemerkung Text"="super geiles PDF", "Align (Left)"=0, "Add Line Feeds (F:No)"=TRUE, "Font"={"Font"="Arial", "Size"=10, "Colour"=0, "Bold"=FALSE, "Italic"=FALSE, "Underline"=FALSE, "Strikethrough"=FALSE, "Font Encoding"=enum."Cp1252, WinANSI"}}, {"Bemerkung Text"="", "Align (Left)"=0, "Add Line Feeds (F:No)"=FALSE, "Font"={"Font"="Arial", "Size"=10, "Colour"=0, "Bold"=FALSE, "Italic"=FALSE, "Underline"=FALSE, "Strikethrough"=FALSE, "Font Encoding"=enum."Cp1252, WinANSI"}}, {"Bemerkung Text"="Tabelle mit optionalen Ergebnissen", "Align (Left)"=3, "Add Line Feeds (F:No)"=FALSE, "Font"={"Font"="Arial", "Size"=10, "Colour"=0, "Bold"=FALSE, "Italic"=FALSE, "Underline"=FALSE, "Strikethrough"=FALSE, "Font Encoding"=enum."Cp1252, WinANSI"}}, {"Bemerkung Text"="Graph geht ab ... ", "Align (Left)"=0, "Add Line Feeds (F:No)"=FALSE, "Font"={"Font"="Arial", "Size"=10, "Colour"=0, "Bold"=FALSE, "Italic"=FALSE, "Underline"=FALSE, "Strikethrough"=FALSE, "Font Encoding"=enum."Cp1252, WinANSI"}}]} ("Content"), "Titel"=w170, "Header Table"=w183, "Table Array"=w186, "Bemerkungen"=w175) -> (w185:T16)
      n102 = Build Array(w159, w182) -> (w176:T35[])
      n103 = call "AddPageContent.vi"("Title Font"=w173, "Column Ratio left"=w184, "error in"=w202, "Graph Array"=w176, "Content"=w185, "Context (Eingang)"=w201) -> ("error out"=w200:errorcluster, "Context (Ausgang)"=w199:refnum<class "Context.lvclass">)  [unwired: 4 in]
      n104 = call "ClosePage.vi"("popup viewer"=TRUE, "Fehler (Eingang, kein Fehler)"=w200, "Context (Eingang)"=w199) -> ("Fehler (Ausgang)"=w167:errorcluster)  [unwired: 8 in]
    }
    frame #3 {
      n105 = disable-structure shown="Deaktiviert" {
        frame Disabled {
          n106 = vi-ref "PDF_Interface_PDF Protokoll EPA1065_308 T90.vi"() -> (w225:refnum<vi>)
          n107 = call "VI Shut Down.vi"("VI Referenz"=w225) -> ()  [unwired: 11 in]
        }
        frame Enabled {
        }
      }
    }
  }
  "error out" <- w2
